vi "cs_isSessionListValid.vi"(8 "error in (no error)":errorcluster, 11 "Array":dbl[][](array[numeric])=[[1.0, 3.0, 4.0, 5.0, 0.0, 0.0, 0.0, 5.0], [1.0, 3.0, 4.0, 5.0, 0.0, 0.0, 0.0, 5.0], [0.0, 6.0, 7.0, 8.0, 0.0, 0.0, 0.0, 5.0], [1.0, 1.0, 2.0, 3.0, 0.0, 0.0, 0.0, 5.0], [0.0, 7.0, 8.0, 9.0, 0.0, 0.0, 0.0, 5.0], [0.0, 7.0, 8.0, 9.0, 0.0, 0.0, 0.0, 5.0], [1.0, 2.0, 3.0, 4.0, 0.0, 0.0, 0.0, 5.0], [1.0, 2.0, 3.0, 4.0, 0.0, 0.0, 0.0, 0.0], [0.0, 5.0, 6.0, 7.0, 0.0, 0.0, 0.0, 0.0], [0.0, 6.0, 7.0, 8.0, 0.0, 0.0, 0.0, 0.0], [1.0, 1.0, 2.0, 3.0, 0.0, 0.0, 0.0, 0.0], [0.0, 5.0, 6.0, 7.0, 0.0, 0.0, 0.0, 0.0]]) -> (0 "error out":errorcluster, 3 "Valid?":bool=TRUE)   [LabVIEW 2013]
uses:
  <vilib>/Utility/error.llb/DialogType.ctl
panel:
  out "Array 2":dbl[](array[numeric])=[0.0, 5.0, 6.0, 7.0, 0.0, 0.0, 0.0, 0.0]
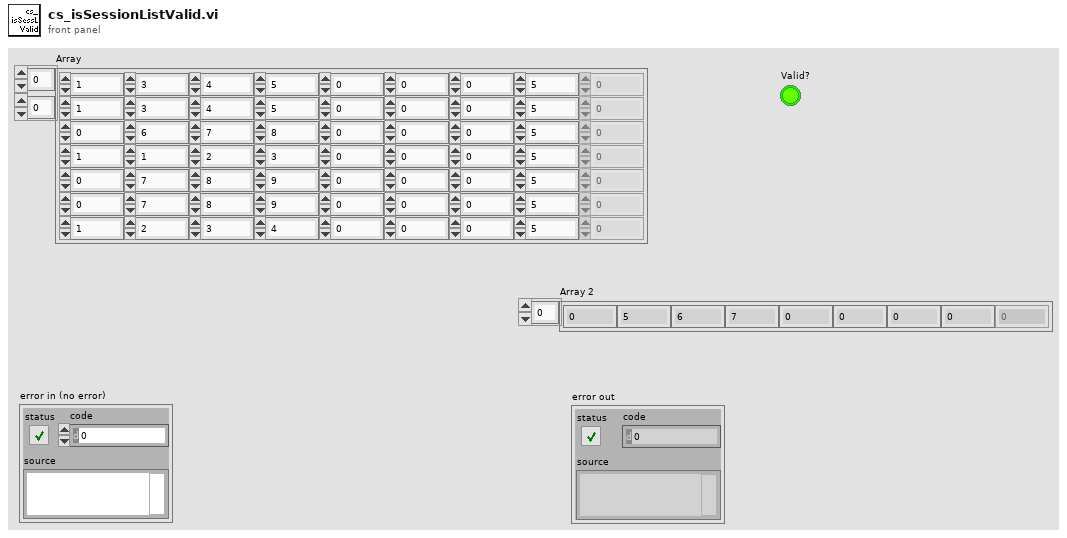
[diagram p1: front panel]
types:
  T1 = typedef "DialogType.ctl" = u16
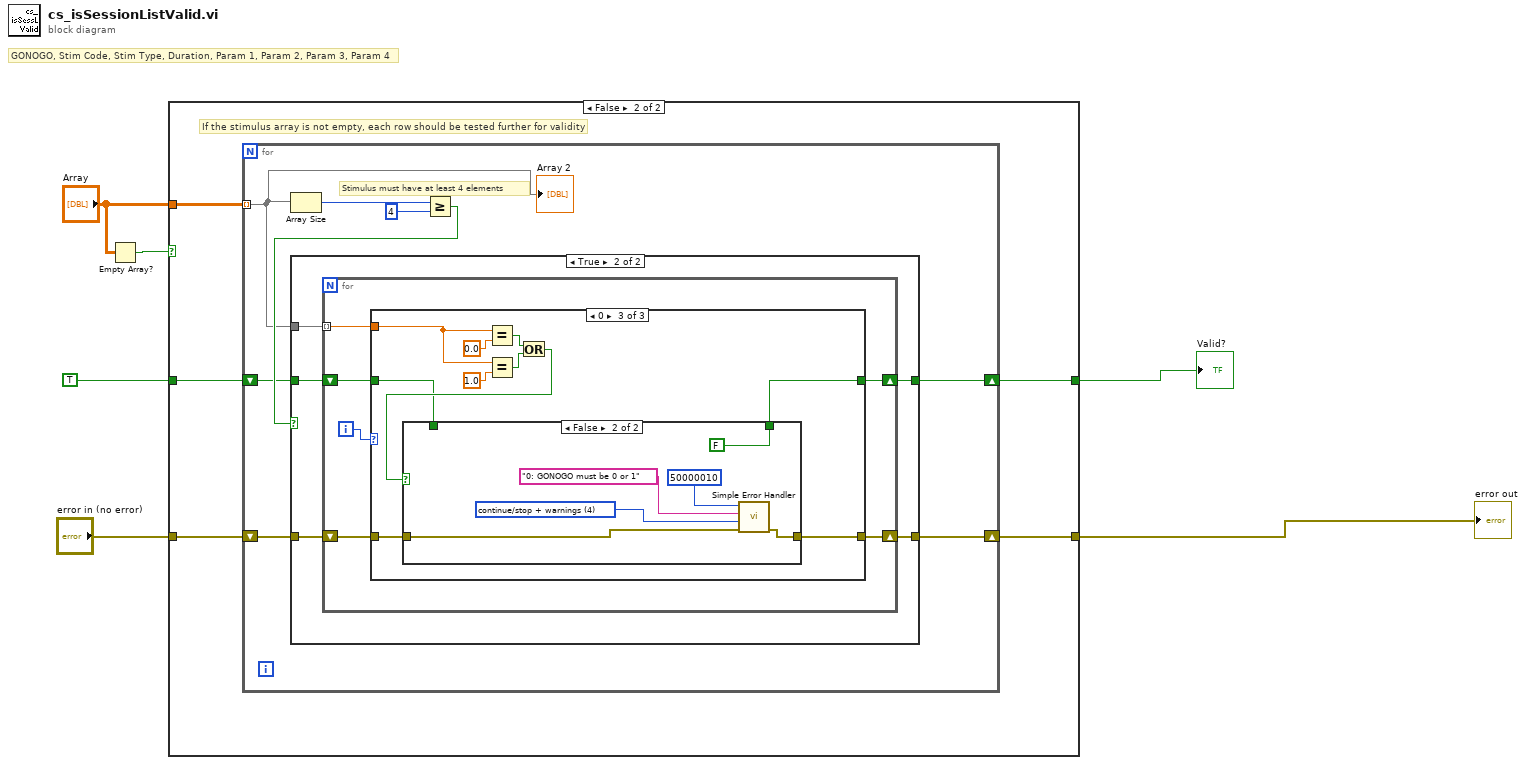
[diagram p0: block diagram]
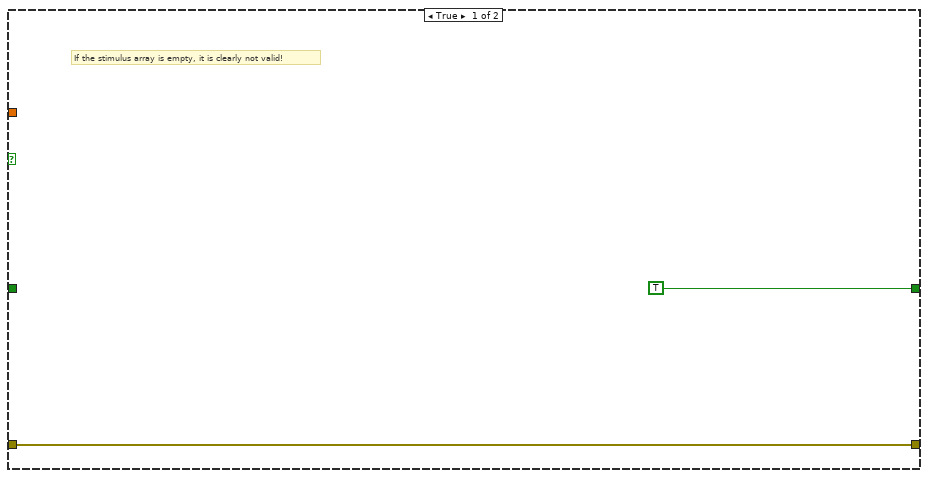
[diagram p2: hidden frame]
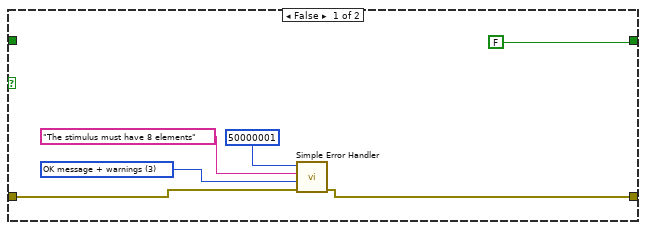
[diagram p3: hidden frame]
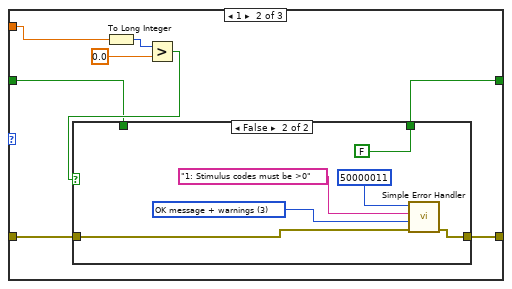
[diagram p5: hidden frame]
diagram:
  # "GONOGO, Stim Code, Stim Type, Duration, Param 1, Param 2, Param 3, Param 4"
  n1 = Empty Array?(array="Array") -> (empty?=w2:bool)
  n2 = case shown="False" w2 {
    tunnel: "Array" -> [_ w13]
    tunnel: "error in (no error)" -> [w7 w12]
    tunnel: [w7 w11] -> w5
    tunnel: TRUE -> [_ w10]
    tunnel: [TRUE w9] -> w3
    frame True {
      # "If the stimulus array is empty, it is clearly not valid!"
    }
    frame False {
      # "If the stimulus array is not empty, each row should be tested further for validity"
      n3 = for {
        tunnel: w13 -> [w14] mode=indexing
        shift-right: [w17] -> w11
        shift-left: w12 -> [w18]
        shift-right: [w15] -> w9
        shift-left: w10 -> [w16]
        # "Stimulus must have at least 4 elements"
        n4 = Array Size(array=w14) -> (size(s)=w20:i32)
        n5 = Greater Or Equal?(x=w20, y=4) -> (x >= y?=w19:bool)
        n6 = case shown="True" w19 {
          tunnel: w14 -> [_ w30]
          tunnel: w18 -> [w27 w32]
          tunnel: [w24 w31] -> w17
          tunnel: w16 -> [_ w29]
          tunnel: [FALSE w28] -> w15
          frame False {
            w26 = T1 3 items=["no dialog", "OK message", "continue or stop message", "OK message + warnings", "continue/stop + warnings"] ("type of dialog (OK msg:1)")
            n7 = call <vilib>:"Simple Error Handler.vi"("error code (no error:0)"=50000001, "error source (\" \")"="The stimulus must have 8 elements" ("error source (\" \")"), "type of dialog (OK msg:1)"=w26, "error in (no error)"=w27) -> ("error out"=w24:errorcluster)  [unwired: 1 in, 4 out]
          }
          frame True {
            n8 = for {
              shift-right: [w36] -> w31
              shift-left: w32 -> [w37]
              tunnel: w30 -> [w38] mode=indexing
              shift-right: [w33] -> w28
              shift-left: w29 -> [w34]
              i -> [w35]
              n9 = case shown="0" w35 {
                tunnel: w38 -> [_ w46 w62]
                tunnel: w37 -> [w40 w44 w61]
                tunnel: [w40 w41 w60] -> w36
                tunnel: w34 -> [w39 w43 w58]
                tunnel: [w39 w42 w57] -> w33
                frame Default {
                }
                frame 1 {
                  n10 = To Long Integer(number=w46) -> (32bit integer=w48:i32)
                  n11 = Greater?(x=w48, y=0.0) -> (0:w45:bool)
                  n12 = case shown="False" w45 {
                    tunnel: w44 -> [w50 w53]
                    tunnel: [w50 w52] -> w41
                    tunnel: w43 -> [w49 _]
                    tunnel: [w49 FALSE] -> w42
                    frame True {
                    }
                    frame False {
                      w56 = T1 3 items=["no dialog", "OK message", "continue or stop message", "OK message + warnings", "continue/stop + warnings"] ("type of dialog (OK msg:1)")
                      n13 = call <vilib>:"Simple Error Handler.vi"("error code (no error:0)"=50000011, "error source (\" \")"="1: Stimulus codes must be >0" ("error source (\" \")"), "type of dialog (OK msg:1)"=w56, "error in (no error)"=w53) -> ("error out"=w52:errorcluster)  [unwired: 1 in, 4 out]
                    }
                  }
                }
                frame 0 {
                  n14 = Equal?(x=w62, y=0.0) -> (x = y?=w65:bool)
                  n15 = Equal?(x=w62, y=1.0) -> (x = y?=w66:bool)
                  n16 = Or(x=w65, y=w66) -> (x .or. y?=w59:bool)
                  n17 = case shown="False" w59 {
                    tunnel: w61 -> [w68 w71]
                    tunnel: [w68 w70] -> w60
                    tunnel: w58 -> [w67 _]
                    tunnel: [w67 FALSE] -> w57
                    frame True {
                    }
                    frame False {
                      w74 = T1 4 items=["no dialog", "OK message", "continue or stop message", "OK message + warnings", "continue/stop + warnings"] ("type of dialog (OK msg:1)")
                      n18 = call <vilib>:"Simple Error Handler.vi"("error code (no error:0)"=50000010, "error source (\" \")"="0: GONOGO must be 0 or 1" ("error source (\" \")"), "type of dialog (OK msg:1)"=w74, "error in (no error)"=w71) -> ("error out"=w70:errorcluster)  [unwired: 1 in, 4 out]
                    }
                  }
                }
              }
            }
          }
        }
        "Array 2" <- w14
      }
    }
  }
  "Valid?" <- w3
  "error out" <- w5
